vi "Get Netway App Version.vi"(0 "Cut-off":string, 11 "Error IN":errorcluster) -> (4 "New Enough?":bool, 6 "Software Installed?":bool, 8 "Current Version":string, 15 "Error OUT":errorcluster)   [LabVIEW 2013]
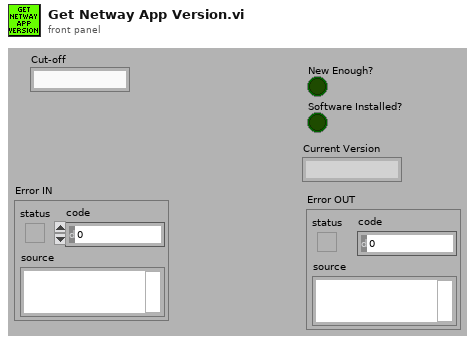
[diagram p1: front panel]
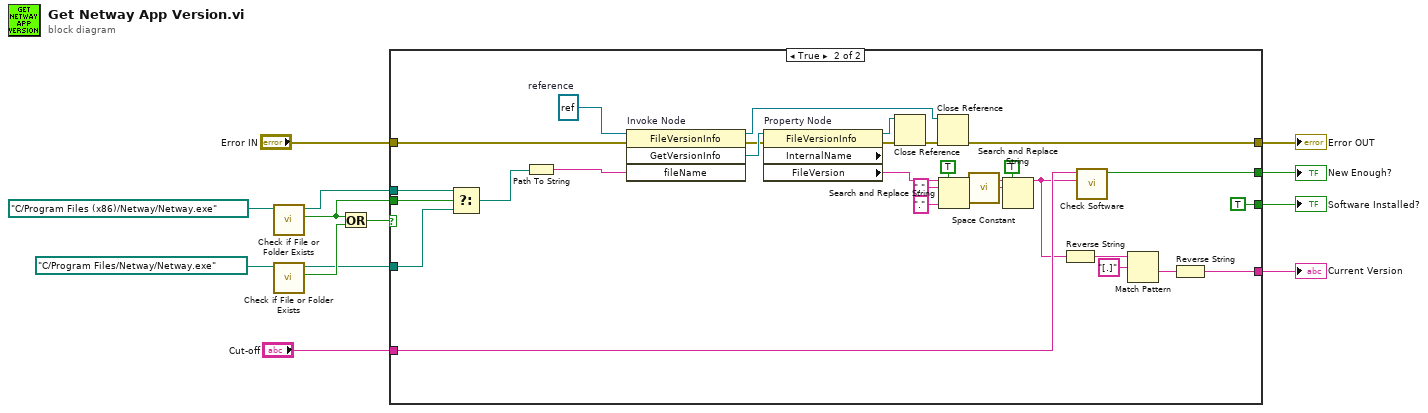
[diagram p0: block diagram]
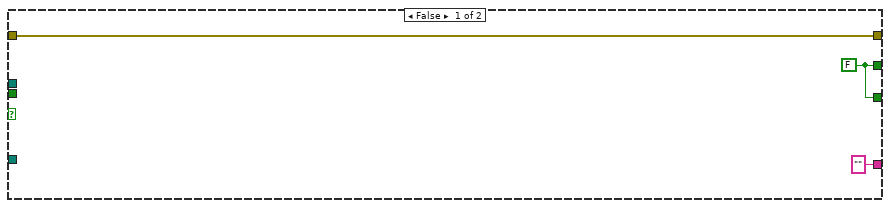
[diagram p2: hidden frame]
diagram:
  n1 = call <vilib>:"Check if File or Folder Exists.vi"("path"=path "C:/Program Files (x86)/Netway/Netway.exe") -> ("file or folder exists?"=w5:bool, "dup path"=w3:path)  [unwired: 8 in, 1 out]
  n2 = call <vilib>:"Check if File or Folder Exists.vi"("path"=path "C:/Program Files/Netway/Netway.exe") -> ("file or folder exists?"=w8:bool, "dup path"=w2:path)  [unwired: 8 in, 1 out]
  n3 = Or(x=w5, y=w8) -> (x .or. y?=w7:bool)
  n4 = case shown="True" w7 {
    tunnel: "Error IN" -> [w16 w37]
    tunnel: [w16 w36] -> w12
    tunnel: "Cut-off" -> [_ w22]
    tunnel: [w15 w32] -> w9
    tunnel: [w15 TRUE ("New Enough?")] -> w6
    tunnel: w5 -> [_ w30]
    tunnel: w3 -> [_ w29]
    tunnel: w2 -> [_ w28]
    tunnel: ["" w18] -> w1
    frame False {
      w15 = FALSE ("New Enough?")
    }
    frame True {
      w45 = refnum<k24> refnum  # reference
      n5 = Select(t=w29, s=w30, f=w28) -> (s? t:f=w27:path)
      n6 = Path To String(path=w27) -> (string=w44:string)
      n7 = invoke on="Invoke Node" class="FileVersionInfo" method="GetVersionInfo"(reference=w45, error in=w37, "fileName"=w44) -> (reference out=w38:refnum<k24>, error out=w42:errorcluster, "GetVersionInfo"=w43:refnum<k24>)  [unwired: 1 in, 1 out]
      n8 = property on="Property Node" class="FileVersionInfo" props=["InternalName", "FileVersion"](reference=w43, error in=w42) -> (reference out=w41:refnum<k24>, error out=w40:errorcluster, "FileVersion"=w26:string)  [unwired: 1 out]
      n9 = Close Reference(reference=w41, error in (no error)=w40) -> (error out=w39:errorcluster)
      n10 = Close Reference(reference=w38, error in (no error)=w39) -> (error out=w36:errorcluster)
      n11 = Search and Replace String(replace all?=TRUE ("replace all? (F)"), input string=w26, search string=",", replace string="." ("replace string (\"\")")) -> (result string=w24:string)  [unwired: 4 in, 3 out]
      n12 = call <vilib>:"Space Constant.vi"() -> ("String"=w23:string)
      n13 = Search and Replace String(replace all?=TRUE ("replace all? (F)"), input string=w24, search string=w23) -> (result string=w17:string)  [unwired: 5 in, 3 out]
      n14 = Reverse String(1:w17) -> (0:w20:string)
      n15 = call "Check Software.vi"("Actual"=w17, "Cut-off"=w22) -> ("New Enough?"=w32:bool)  [unwired: 9 in]
      n16 = Match Pattern(string=w20, regular expression="[.]") -> (after substring=w19:string)  [unwired: 1 in, 3 out]
      n17 = Reverse String(1:w19) -> (0:w18:string)
    }
  }
  "Error OUT" <- w12
  "New Enough?" <- w9
  "Software Installed?" <- w6
  "Current Version" <- w1
